vi "ReadLoop.vi"(1 "lines":u32, 2 "exttrig":u32=5, 3 "pixel":u32=1, 4 "threadp":u32=5, 5 "freq":u32, 6 "exptus":u32=20000, 7 "nos":u32=1) -> (0 "Data Values":u32[][](graph))   [LabVIEW 2014]
uses:
  ESLSCDLL.dll
panel:
  in  "clrcnt":u32=8
  in  "zadr":u32=1
  in  "lfkt":i32=1
  # "lines for  FFTs, or 0 else"
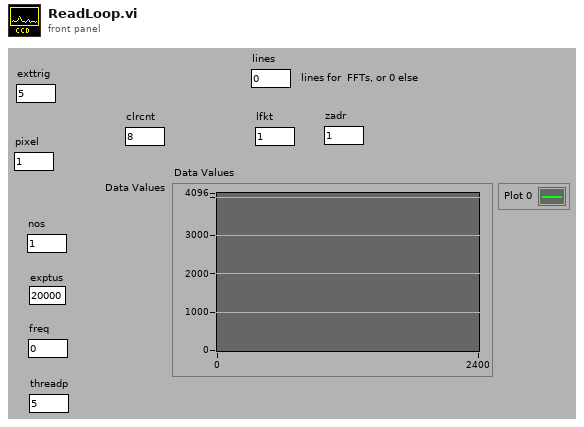
[diagram p1: front panel]
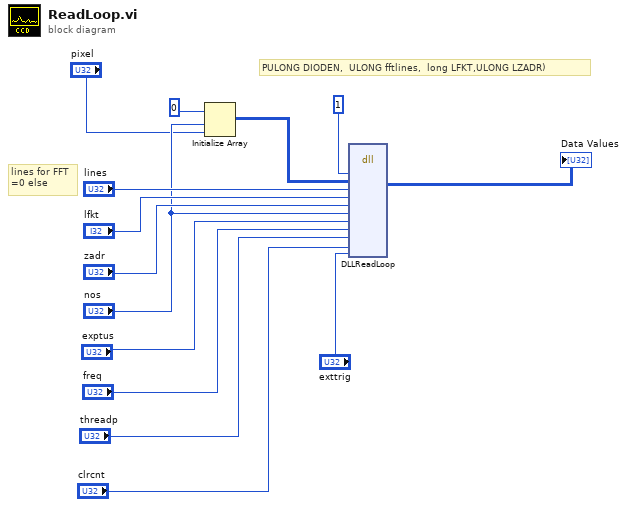
[diagram p0: block diagram]
diagram:
  # "lines for FFT\n=0 else"
  # "PULONG DIODEN, \tULONG fftlines,  long LFKT,ULONG LZADR)"
  n1 = Initialize Array(u32 0, "nos", "pixel") -> (w2:u32[][])
  n2 = dll-call lib="C:/Users/Gerhard/Documents/New64/lv/1cam/board.vis/ESLSCDLL.dll" fn="DLLReadLoop"("drv"=u32 1, "dioden"=w2, "fftlines"="lines", "fkt"="lfkt", "zadr"="zadr", "nos"="nos", "exptus"="exptus", "freq"="freq", "threadp"="threadp", "clrcnt"="clrcnt", "exttrig"="exttrig") -> ("dioden"=→"Data Values":u32[][])  [unwired: 14 in, 2 out]
